vi "Wait.vi"(6 "Reset":bool, 11 "milliseconds to wait":i32) -> (3 "Finished":bool)   [LabVIEW 2018, in "ArduinoSerialBling.lvlib"]
uses:
  ArduinoSerialBling.lvlib
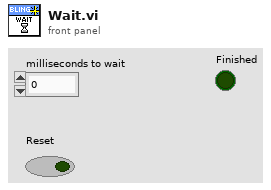
[diagram p1: front panel]
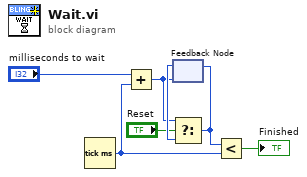
[diagram p0: block diagram]
diagram:
  n1 = Tick Count (ms)() -> (millisecond timer value=w4:u32)
  n2 = Add(x="milliseconds to wait", y=w4) -> (x+y=w5:u32)
  n3 = feedback #1(w5) -> (w6:u32)
  n4 = Select(t=w5, s="Reset", f=w6) -> (s? t:f=w1:u32)
  n5 = feedback-in #1(w1) -> ()
  n6 = Less?(x=w1, y=w4) -> (x < y?=→"Finished":bool)
